vi "SP Get Data Channels From Plot.vi"(8 "error in (no error)":errorcluster, 9 "Plot Ref":refnum<vi>) -> (0 "error out":errorcluster, 2 "CH 2":T1, 3 "CH 1":T1)   [LabVIEW 2011]
uses:
  TypeDefs/SP Channel Data.ctl
  TypeDefs/SP Plot Cluster Object.ctl
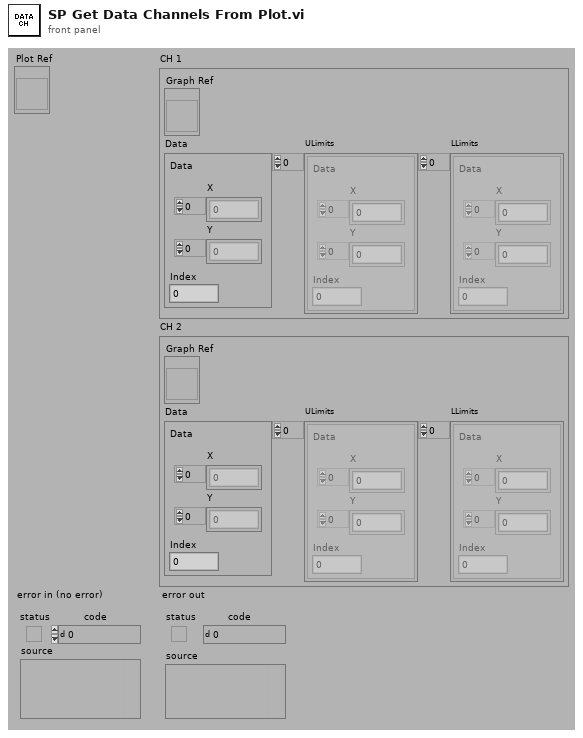
[diagram p1: front panel]
types:
  T1 = typedef "SP Channel Data.ctl" = cluster{"Graph Ref":refnum<vi>, "Data":cluster{"Data":cluster{"X":dbl[], "Y":dbl[]}, "Index":i32}, "ULimits":cluster{"Data":cluster{"X":dbl[], "Y":dbl[]}, "Index":i32}[], "LLimits":cluster{"Data":cluster{"X":dbl[], "Y":dbl[]}, "Index":i32}[]}
  T2 = cluster{"Data":cluster{"X":dbl[], "Y":dbl[]}, "Index":i32}
  T3 = typedef "SP Plot Cluster Object.ctl" = enum16{"Plot", "CH Reference", "CH Label", "Start Label", "Stop Label", "Units Label", "Selected?", "CH Markers"}
  T4 = cluster{"Data":cluster{"X":dbl[], "Y":dbl[]}, "Index":i32}[]
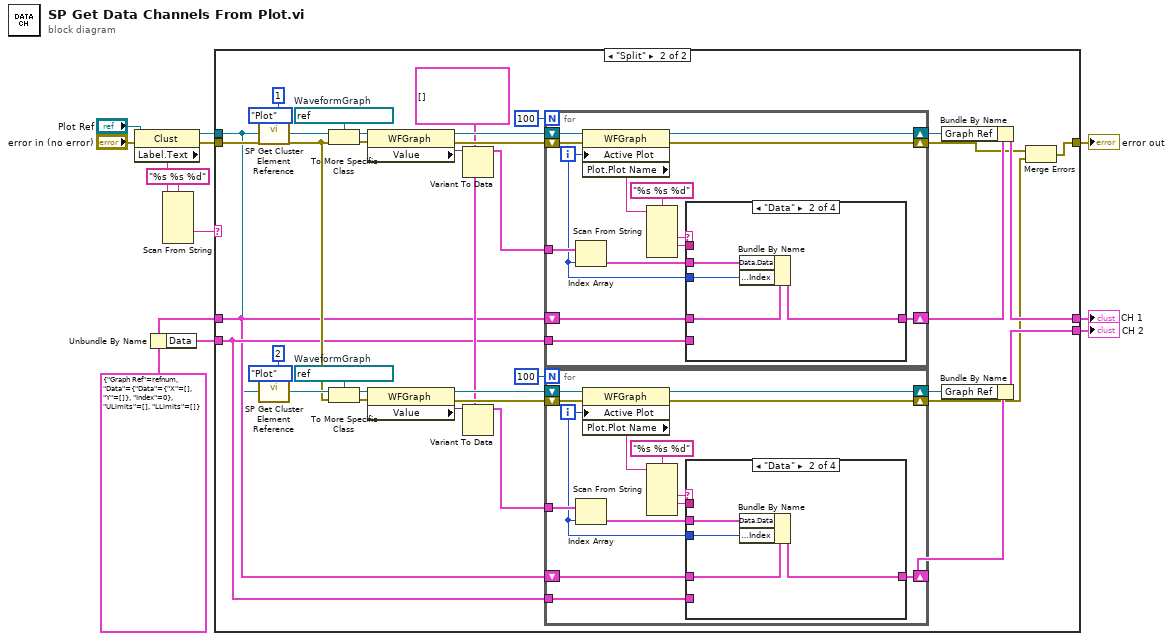
[diagram p0: block diagram]
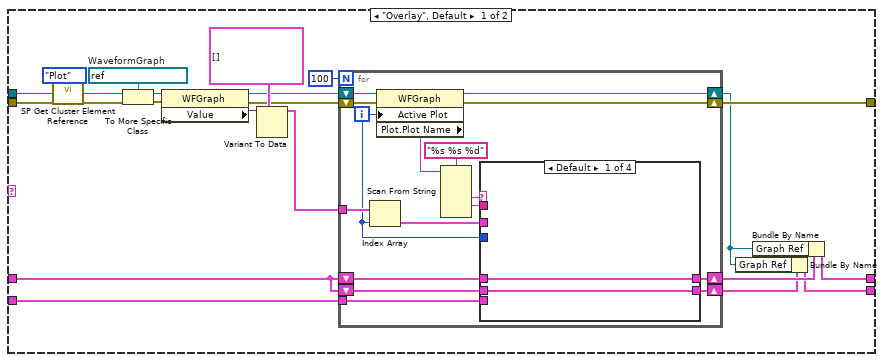
[diagram p2: hidden frame]
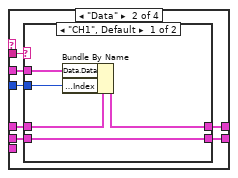
[diagram p3: hidden frame]
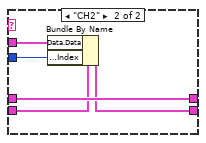
[diagram p4: hidden frame]
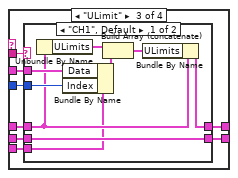
[diagram p5: hidden frame]
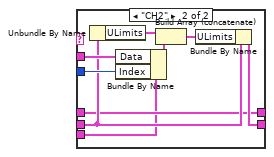
[diagram p6: hidden frame]
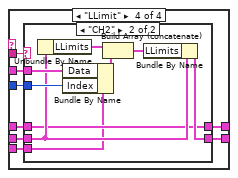
[diagram p7: hidden frame]
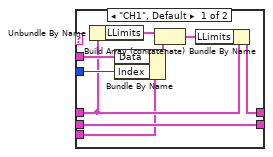
[diagram p8: hidden frame]
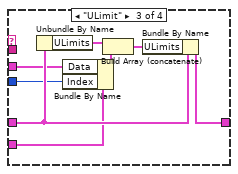
[diagram p10: hidden frame]
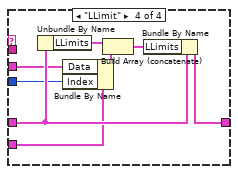
[diagram p11: hidden frame]
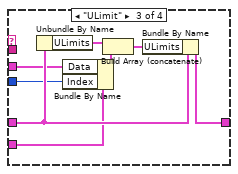
[diagram p13: hidden frame]
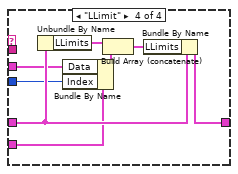
[diagram p14: hidden frame]
diagram:
  w1 = T1 {"Graph Ref"=refnum, "Data"={"Data"={"X"=[], "Y"=[]}, "Index"=0}, "ULimits"=[], "LLimits"=[]} ("CH")
  n1 = property class="Clust"(reference="Plot Ref", error in="error in (no error)") -> (reference out=w7:refnum<vi>, error out=w8:errorcluster, "Label.Text"=w11:string)
  n2 = Unbundle By Name(w1) -> ("Data"=w2:T2)
  n3 = Scan From String(format string="%s %s %d", input string=w11) -> (output 2=w9:string)  [unwired: 2 in, 8 out]
  n4 = case shown="\"Split\"" w9 {
    tunnel: w8 -> [w14 w133]
    tunnel: [w23 w124] -> w6
    tunnel: w7 -> [w27 w121]
    tunnel: [w18 w127] -> w3
    tunnel: [w20 w146] -> w4
    tunnel: w2 -> [w16 w129]
    tunnel: w1 -> [w15 w128]
    frame "Overlay", Default {
      w31 = refnum<vi> refnum  # WaveformGraph
      n5 = call "SP Get Cluster Element Reference.vi"("Element"=SP_Plot_Cluster_Object."Plot", "Plot Reference"=w27) -> ("Element Reference"=w32:refnum<vi>)  [unwired: 1 in, 6 out]
      n6 = To More Specific Class(target class=w31, reference=w32, error in=w14) -> (specific class reference=w26:refnum<vi>, error out=w13:errorcluster)
      n7 = property class="WFGraph"(reference=w26, error in=w13) -> (reference out=w24:refnum<vi>, error out=w25:errorcluster, "Value"=w28:variant)
      n8 = Variant To Data(type=cluster{"X":dbl[], "Y":dbl[]}[] [] ("appended array"), Variant=w28) -> (data=w22:cluster{"X":dbl[], "Y":dbl[]}[])  [unwired: 1 in, 1 out]
      n9 = for {
        N: 100 -> [_]
        shift-right: [w47] -> w23
        shift-left: w25 -> [w46]
        shift-right: [w48] -> w17
        shift-left: w24 -> [w49]
        shift-right: [w41] -> w21
        shift-left: w15 -> [w38]
        shift-right: [w40] -> w19
        shift-left: w15 -> [w39]
        tunnel: w22 -> [w37]
        tunnel: w16 -> [w34]
        i -> [w35]
        n10 = Index Array(array=w37, index=w35) -> (element=w36:cluster{"X":dbl[], "Y":dbl[]})
        n11 = property class="WFGraph"(reference=w49, error in=w46, "Active Plot"=w35) -> (reference out=w48:refnum<vi>, error out=w47:errorcluster, "Plot.Plot Name"=w44:string)
        n12 = Scan From String(format string="%s %s %d", input string=w44) -> (output 1=w43:string, output 2=w42:string)  [unwired: 2 in, 7 out]
        n13 = case shown="Default" w43 {
          tunnel: w42 -> [_ w58 w76 w102]
          tunnel: [w50 w57 w71 w97] -> w41
          tunnel: [w51 w56 w70 w96] -> w40
          tunnel: w39 -> [w51 w55 w75 w101]
          tunnel: w38 -> [w50 w54 w74 w100]
          tunnel: w36 -> [_ w53 w73 w99]
          tunnel: w35 -> [_ w52 w72 w98]
          tunnel: w34 -> [_ _ w69 w95]
          frame Default {
          }
          frame "Data" {
            n14 = case shown="\"CH1\", Default" w58 {
              tunnel: [w59 w66] -> w57
              tunnel: [w63 w64] -> w56
              tunnel: w55 -> [w63 w65]
              tunnel: w54 -> [w62 w66]
              tunnel: w53 -> [w61 w68]
              tunnel: w52 -> [w60 w67]
              frame "CH1", Default {
                n15 = Bundle By Name(cluster=w62, "Data.Data"=w61, "Data.Index"=w60) -> (w59:T1)
              }
              frame "CH2" {
                n16 = Bundle By Name(cluster=w65, "Data.Data"=w68, "Data.Index"=w67) -> (w64:T1)
              }
            }
          }
          frame "ULimit" {
            n17 = case shown="\"CH1\", Default" w76 {
              tunnel: w75 -> [w78 w88]
              tunnel: w74 -> [w81 w87]
              tunnel: w73 -> [w84 w93]
              tunnel: w72 -> [w83 w92]
              tunnel: [w79 w87] -> w71
              tunnel: [w78 w89] -> w70
              tunnel: w69 -> [w77 w86]
              frame "CH1", Default {
                n18 = Unbundle By Name(w81) -> ("ULimits"=w85:T4)
                n19 = Bundle By Name(cluster=w77, "Data"=w84, "Index"=w83) -> (w82:T2)
                n20 = Build Array (concatenate)(w85, w82) -> (w80:T4)
                n21 = Bundle By Name(cluster=w81, "ULimits"=w80) -> (w79:T1)
              }
              frame "CH2" {
                n22 = Unbundle By Name(w88) -> ("ULimits"=w94:T4)
                n23 = Bundle By Name(cluster=w86, "Data"=w93, "Index"=w92) -> (w91:T2)
                n24 = Build Array (concatenate)(w94, w91) -> (w90:T4)
                n25 = Bundle By Name(cluster=w88, "ULimits"=w90) -> (w89:T1)
              }
            }
          }
          frame "LLimit" {
            n26 = case shown="\"CH2\"" w102 {
              tunnel: w101 -> [w104 w114]
              tunnel: w100 -> [w107 w113]
              tunnel: w99 -> [w110 w119]
              tunnel: w98 -> [w109 w118]
              tunnel: [w105 w113] -> w97
              tunnel: [w104 w115] -> w96
              tunnel: w95 -> [w103 w112]
              frame "CH1", Default {
                n27 = Unbundle By Name(w107) -> ("LLimits"=w111:T4)
                n28 = Bundle By Name(cluster=w103, "Data"=w110, "Index"=w109) -> (w108:T2)
                n29 = Build Array (concatenate)(w111, w108) -> (w106:T4)
                n30 = Bundle By Name(cluster=w107, "LLimits"=w106) -> (w105:T1)
              }
              frame "CH2" {
                n31 = Unbundle By Name(w114) -> ("LLimits"=w120:T4)
                n32 = Bundle By Name(cluster=w112, "Data"=w119, "Index"=w118) -> (w117:T2)
                n33 = Build Array (concatenate)(w120, w117) -> (w116:T4)
                n34 = Bundle By Name(cluster=w114, "LLimits"=w116) -> (w115:T1)
              }
            }
          }
        }
      }
      n35 = Bundle By Name(cluster=w19, "Graph Ref"=w17) -> (w18:T1)
      n36 = Bundle By Name(cluster=w21, "Graph Ref"=w17) -> (w20:T1)
    }
    frame "Split" {
      w136 = refnum<vi> refnum  # WaveformGraph
      w130 = cluster{"X":dbl[], "Y":dbl[]}[] [] ("appended array")
      w154 = refnum<vi> refnum  # WaveformGraph
      n37 = call "SP Get Cluster Element Reference.vi"("Channel"=i8 1, "Element"=SP_Plot_Cluster_Object."Plot", "Plot Reference"=w121) -> ("Element Reference"=w155:refnum<vi>)  [unwired: 6 out]
      n38 = call "SP Get Cluster Element Reference.vi"("Channel"=i8 2, "Element"=SP_Plot_Cluster_Object."Plot", "Plot Reference"=w121) -> ("Element Reference"=w135:refnum<vi>)  [unwired: 6 out]
      n39 = To More Specific Class(target class=w154, reference=w155, error in=w133) -> (specific class reference=w151:refnum<vi>, error out=w132:errorcluster)
      n40 = To More Specific Class(target class=w136, reference=w135, error in=w133) -> (specific class reference=w139:refnum<vi>, error out=w131:errorcluster)
      n41 = property class="WFGraph"(reference=w151, error in=w132) -> (reference out=w149:refnum<vi>, error out=w150:errorcluster, "Value"=w152:variant)
      n42 = property class="WFGraph"(reference=w139, error in=w131) -> (reference out=w141:refnum<vi>, error out=w140:errorcluster, "Value"=w138:variant)
      n43 = Variant To Data(type=w130, Variant=w152) -> (data=w148:cluster{"X":dbl[], "Y":dbl[]}[])  [unwired: 1 in, 1 out]
      n44 = Variant To Data(type=w130, Variant=w138) -> (data=w142:cluster{"X":dbl[], "Y":dbl[]}[])  [unwired: 1 in, 1 out]
      n45 = for {
        N: 100 -> [_]
        shift-right: [w203] -> w125
        shift-left: w150 -> [w202]
        shift-right: [w204] -> w145
        shift-left: w149 -> [w205]
        shift-right: [w197] -> w147
        shift-left: w128 -> [w196]
        tunnel: w148 -> [w195]
        tunnel: w129 -> [w192]
        i -> [w193]
        n46 = Index Array(array=w195, index=w193) -> (element=w194:cluster{"X":dbl[], "Y":dbl[]})
        n47 = property class="WFGraph"(reference=w205, error in=w202, "Active Plot"=w193) -> (reference out=w204:refnum<vi>, error out=w203:errorcluster, "Plot.Plot Name"=w200:string)
        n48 = Scan From String(format string="%s %s %d", input string=w200) -> (output 1=w199:string, output 2=w198:string)  [unwired: 2 in, 7 out]
        n49 = case shown="\"Data\"" w199 {
          tunnel: w198 -> [_ _ _ _]
          tunnel: [w206 w210 w214 w222] -> w197
          tunnel: w196 -> [w206 w209 w218 w226]
          tunnel: w194 -> [_ w208 w216 w224]
          tunnel: w193 -> [_ w207 w215 w223]
          tunnel: w192 -> [_ _ w217 w225]
          frame Default {
          }
          frame "Data" {
            n50 = Bundle By Name(cluster=w209, "Data.Data"=w208, "Data.Index"=w207) -> (w210:T1)
          }
          frame "ULimit" {
            n51 = Unbundle By Name(w218) -> ("ULimits"=w213:T4)
            n52 = Bundle By Name(cluster=w217, "Data"=w216, "Index"=w215) -> (w212:T2)
            n53 = Build Array (concatenate)(w213, w212) -> (w211:T4)
            n54 = Bundle By Name(cluster=w218, "ULimits"=w211) -> (w214:T1)
          }
          frame "LLimit" {
            n55 = Unbundle By Name(w226) -> ("LLimits"=w221:T4)
            n56 = Bundle By Name(cluster=w225, "Data"=w224, "Index"=w223) -> (w220:T2)
            n57 = Build Array (concatenate)(w221, w220) -> (w219:T4)
            n58 = Bundle By Name(cluster=w226, "LLimits"=w219) -> (w222:T1)
          }
        }
      }
      n59 = for {
        N: 100 -> [_]
        shift-right: [w168] -> w126
        shift-left: w140 -> [w167]
        shift-right: [w169] -> w144
        shift-left: w141 -> [w170]
        shift-right: [w162] -> w143
        shift-left: w128 -> [w161]
        tunnel: w142 -> [w160]
        tunnel: w129 -> [w157]
        i -> [w158]
        n60 = Index Array(array=w160, index=w158) -> (element=w159:cluster{"X":dbl[], "Y":dbl[]})
        n61 = property class="WFGraph"(reference=w170, error in=w167, "Active Plot"=w158) -> (reference out=w169:refnum<vi>, error out=w168:errorcluster, "Plot.Plot Name"=w165:string)
        n62 = Scan From String(format string="%s %s %d", input string=w165) -> (output 1=w164:string, output 2=w163:string)  [unwired: 2 in, 7 out]
        n63 = case shown="\"Data\"" w164 {
          tunnel: w163 -> [_ _ _ _]
          tunnel: [w171 w175 w179 w187] -> w162
          tunnel: w161 -> [w171 w174 w183 w191]
          tunnel: w159 -> [_ w173 w181 w189]
          tunnel: w158 -> [_ w172 w180 w188]
          tunnel: w157 -> [_ _ w182 w190]
          frame Default {
          }
          frame "Data" {
            n64 = Bundle By Name(cluster=w174, "Data.Data"=w173, "Data.Index"=w172) -> (w175:T1)
          }
          frame "ULimit" {
            n65 = Unbundle By Name(w183) -> ("ULimits"=w178:T4)
            n66 = Bundle By Name(cluster=w182, "Data"=w181, "Index"=w180) -> (w177:T2)
            n67 = Build Array (concatenate)(w178, w177) -> (w176:T4)
            n68 = Bundle By Name(cluster=w183, "ULimits"=w176) -> (w179:T1)
          }
          frame "LLimit" {
            n69 = Unbundle By Name(w191) -> ("LLimits"=w186:T4)
            n70 = Bundle By Name(cluster=w190, "Data"=w189, "Index"=w188) -> (w185:T2)
            n71 = Build Array (concatenate)(w186, w185) -> (w184:T4)
            n72 = Bundle By Name(cluster=w191, "LLimits"=w184) -> (w187:T1)
          }
        }
      }
      n73 = Bundle By Name(cluster=w147, "Graph Ref"=w145) -> (w146:T1)
      n74 = Bundle By Name(cluster=w143, "Graph Ref"=w144) -> (w127:T1)
      n75 = Merge Errors(w125, w126) -> (w124:errorcluster)
    }
  }
  "CH 2" <- w3
  "error out" <- w6
  "CH 1" <- w4
